vi "drawRectangle.vi"(0 "reference":refnum<class "Graphics.lvclass">, 1 "rectangle":T1 {"height" format="%.2f"; "width" format="%.2f"; "y" format="%.2f"; "x" format="%.2f"}, 2 "lineWidth(1)":dbl=1.0 format="%.2f", 3 "color(if not used=default color)":u32=33554432 format="%.0x", 4 "fill?(F)":bool, 5 "error in (no error)":errorcluster, 7 "FillClor(if not used=BorderColorIsUsed,AutoFill)":u32=16777216 format="%.0x") -> (14 "reference out":refnum<class "Graphics.lvclass">, 19 "error out":errorcluster)   [LabVIEW 2016, in "Graphics.lvclass"]
doc: "Draws a rectangle"
uses:
  <resource>/Framework/Providers/Open_GDS/UML/Graphics_class/Graphics.lvclass
  <resource>/Framework/Providers/Open_GDS/UML/General/Rectangle/Rectangle Rectangle2D.ctl
panel:
  # "Always set\nVI Server class\nto current VI. Do not\nconnect this control\nto the connector pane.\n(Tip!: Just drag\nand drop the icon\ninto the refnum)"
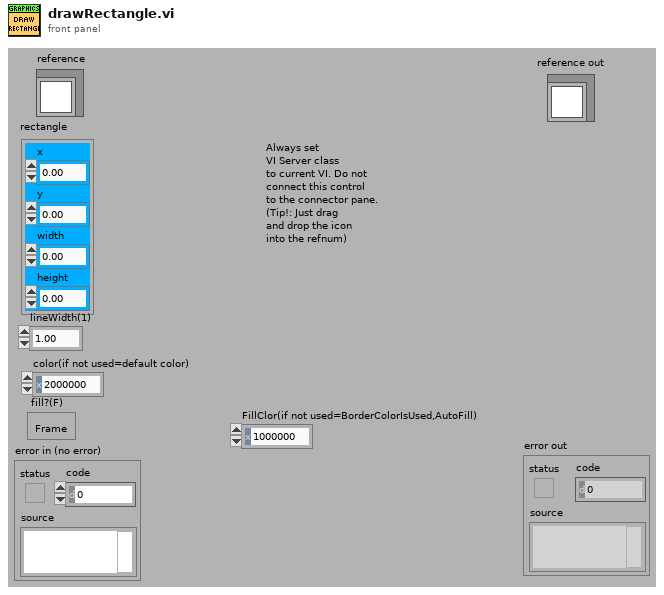
[diagram p1: front panel]
types:
  T1 = typedef "Rectangle Rectangle2D.ctl" = cluster{"x":dbl, "y":dbl, "width":dbl, "height":dbl}
  T2 = cluster{"Width":i16, "Style":enum32{"Solid", "Dash", "Dot", "DashDot", "DashDotDot"}}
  T3 = typedef "Graphics.lvclass/ObjectAttributes.ctl" = cluster{"drawColor":u32, "backgroundColor":u32, "font":T4, "fontType":T5, "picture":picture, "stroke":T6, "scaleX":dbl, "scaleY":dbl, "screenRef":refnum<vi>, "offsetX":dbl, "offsetY":dbl}
  T4 = typedef "Graphics.lvclass/FontType.ctl" = cluster{"Font Name:":string, "Size":i16, "Strikeout?":bool, "Italic?":bool, "Underline?":bool, "Outline?":bool, "Shadow?":bool, "Bold?":bool}
  T5 = typedef "Graphics.lvclass/LvFontType.ctl" = enum16{"User-specified Font", "Application Font", "System Font", "Dialog Font"}
  T6 = typedef "Graphics.lvclass/StrokeType.ctl" = enum16{"USE_DEFAULT", "SOLID", "DOTTED"}
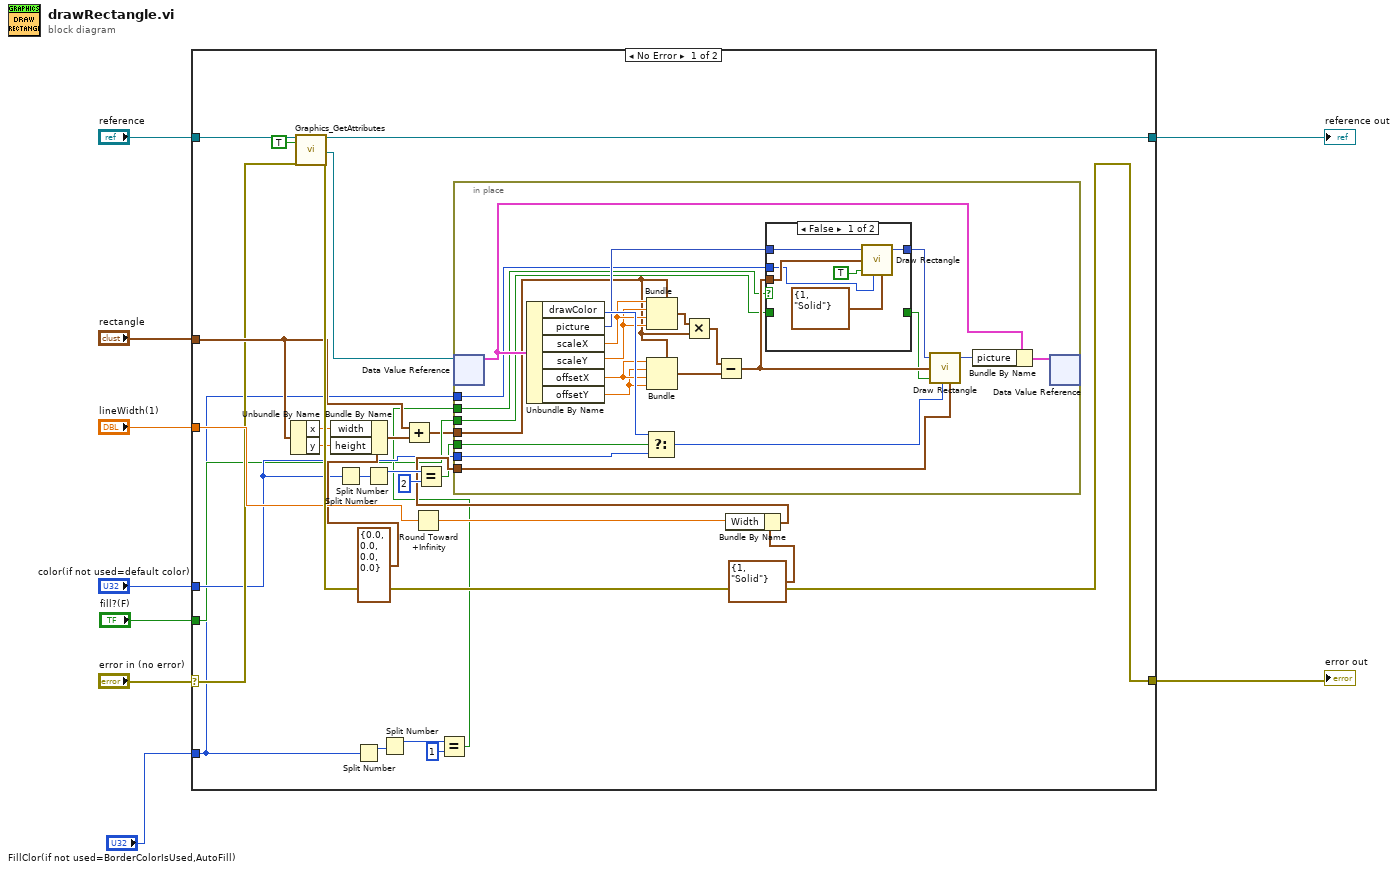
[diagram p0: block diagram]
diagram:
  n1 = case shown="No Error" "error in (no error)" {
    selector: "error in (no error)" -> [w31 w68]
    tunnel: "reference" -> [w36 w69]
    tunnel: [w35 w68] -> w8
    tunnel: [w34 w69] -> w7
    tunnel: "rectangle" -> [w33 _]
    tunnel: "lineWidth(1)" -> [w32 _]
    tunnel: "color(if not used=default color)" -> [w15 _]
    tunnel: "fill?(F)" -> [w12 _]
    tunnel: "FillClor(if not used=BorderColorIsUsed,AutoFill)" -> [w11 _]
    frame No Error {
      n2 = Unbundle By Name(w33) -> ("x"=w26:dbl, "y"=w25:dbl)
      n3 = call <resource>:"Graphics_GetAttributes.vi"("reference in"=w36, "OnlyGetDvrReference(False)"=TRUE, "error in (no error)"=w31) -> ("reference out"=w34:refnum<class "Graphics.lvclass">, "DataRef"=w17:refnum<data-value>, "error out"=w35:errorcluster)  [unwired: 13 in, 1 out]
      n4 = Bundle By Name(cluster=T1 {"x"=0.0, "y"=0.0, "width"=0.0, "height"=0.0} ("x"), "width"=w26, "height"=w25) -> (w24:T1)
      n5 = Split Number(x=w15) -> (hi(x)=w30:u16)  [unwired: 1 out]
      n6 = Split Number(x=w11) -> (hi(x)=w21:u16)  [unwired: 1 out]
      n7 = Split Number(x=w30) -> (hi(x)=w29:u8)  [unwired: 1 out]
      n8 = Split Number(x=w21) -> (hi(x)=w22:u8)  [unwired: 1 out]
      n9 = Add(x=w33, y=w24) -> (x+y=w10:T1)
      n10 = Round Toward +Infinity(x=w32) -> (ceil(x): smallest int >= x=w19:dbl)
      n11 = Equal?(x=w29, y=u8 2) -> (x = y?=w14:bool)
      n12 = Equal?(x=w22, y=u8 1) -> (x = y?=w13:bool)
      n13 = Bundle By Name(cluster=T2 {"Width"=1, "Style"=enum."Solid"} ("pen"), "Width"=w19) -> (w16:T2)
      n14 = in-place {
        in-place-border: w16 -> [w46]
        in-place-border: w15 -> [w45]
        in-place-border: w14 -> [w44]
        in-place-border: w13 -> [w43]
        in-place-border: w12 -> [w42]
        in-place-border: w11 -> [w41]
        in-place-border: w10 -> [w37]
        n15 = in-place-dvr #1(w17) -> (w59:T3)  [unwired: 1 out]
        n16 = Unbundle By Name(w59) -> ("drawColor"=w56:u32, "picture"=w55:picture, "scaleX"=w54:dbl, "scaleY"=w53:dbl, "offsetX"=w52:dbl, "offsetY"=w51:dbl)
        n17 = Select(t=w56, s=w44, f=w45) -> (s? t:f=w47:u32)
        n18 = Bundle(cluster=w37, "x"=w54, "y"=w53, "width"=w54, "height"=w53) -> (w40:T1)
        n19 = Bundle(cluster=w37, "x"=w52, "y"=w51, "width"=w52, "height"=w51) -> (w39:T1)
        n20 = Multiply(x=w40, y=w37) -> (x*y=w38:T1)
        n21 = Subtract(x=w38, y=w39) -> (x-y=w49:T1)
        n22 = case shown="False" w43 {
          tunnel: w42 -> [_ w67]
          tunnel: [_ w67] -> w48
          tunnel: w55 -> [w65 w66]
          tunnel: [w64 w66] -> w50
          tunnel: w49 -> [w63 _]
          tunnel: w41 -> [w62 _]
          frame False {
            n23 = call <vilib>:"Draw Rectangle.vi"("picture"=w65, "rect"=w63, "fill?(F)"=TRUE, "color(black)"=w62, "pen"=T2 {"Width"=1, "Style"=enum."Solid"}) -> ("new picture"=w64:picture)  [unwired: 4 in]
          }
          frame True {
          }
        }
        n24 = call <vilib>:"Draw Rectangle.vi"("picture"=w50, "rect"=w49, "fill?(F)"=w48, "color(black)"=w47, "pen"=w46) -> ("new picture"=w58:picture)  [unwired: 4 in]
        n25 = Bundle By Name(cluster=w59, "picture"=w58) -> (w57:T3)
        n26 = in-place-dvr #1(w57) -> ()  [unwired: 2 out]
      }
    }
    frame Error {
    }
  }
  "reference out" <- w7
  "error out" <- w8
